vi "Connect to PS3 Controller.vi"() -> (0 "error out":errorcluster, 2 "device ID 2":refnum<k1>)   [LabVIEW 2014]
panel:
  out "ID":i32
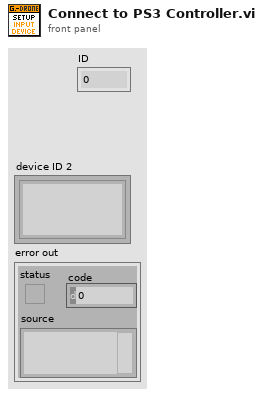
[diagram p1: front panel]
types:
  T1 = cluster{"axes total":u32, "buttons total":u32, "pov total":u32, "device name":string}[]
  T2 = cluster{"axes total":u32, "buttons total":u32, "pov total":u32, "device name":string}
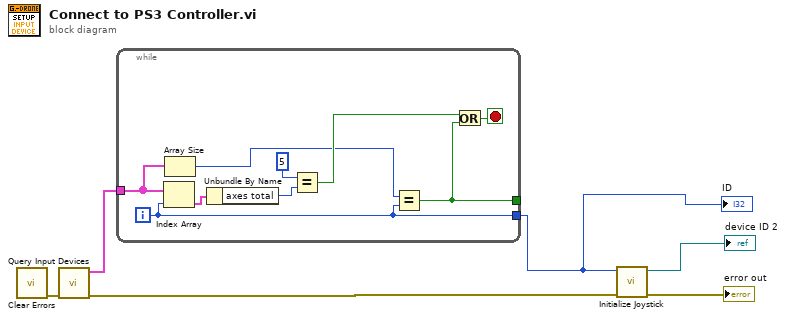
[diagram p0: block diagram]
diagram:
  n1 = call <vilib>:"Clear Errors.vi"() -> ("error out"=w2:errorcluster)  [unwired: 6 in, 1 out]
  n2 = call <vilib>:"Query Input Devices.vi"("error in (no error)"=w2) -> ("error out"=w4:errorcluster, "joystick info"=w6:T1)  [unwired: 7 in, 2 out]
  n3 = while {
    tunnel: w6 -> [w9]
    tunnel: [w10] -> w1
    tunnel: [w8] -> _
    i -> [w10]
    stop <- w12 stop-if-true
    n4 = Index Array(array=w9, index=w10) -> (element=w15:T2)
    n5 = Array Size(array=w9) -> (size(s)=w7:i32)
    n6 = Unbundle By Name(w15) -> ("axes total"=w13:u32)
    n7 = Equal?(x=u32 5 ("y"), y=w13) -> (x = y?=w11:bool)
    n8 = Equal?(x=w7, y=w10) -> (x = y?=w8:bool)
    n9 = Or(x=w11, y=w8) -> (x .or. y?=w12:bool)
  }
  "ID" <- w1
  n10 = call <vilib>:"Initialize Joystick.vi"("error in (no error)"=w4, "device index"=w1) -> ("error out"=→"error out":errorcluster, "device ID"=→"device ID 2":refnum<k1>)  [unwired: 8 in]
